vi "1.1 PID Squared .vi"(9 "2.1 PID Gains":T1={"P Gain"=0.25, "I Gain"=0.9999923706054688, "D Gain"=0.0, "P Gain - Exp"=2, "I Gain - Exp"=2, "D Gain - Exp"=2, "I Saturate"=0.25} {"I Saturate" format="%#_14g"; "P Gain" format="%.8f"; "I Gain" format="%.8f"; "D Gain" format="%.8f"}, 10 "Setpoint":i32, 11 "Encoder Value":i32) -> (0 "D Error":fxp<+/-,18,1> format="%.18g", 1 "I Error":fxp<+/-,64,46> format="%.32g", 2 "Analog Output":fxp<+/-,20,5> format="%.17g", 4 "Error":fxp<+/-,18,1> format="%.18g")   [LabVIEW 2010]
doc: "PID controll for FPGA (fixed point math) without the \"I\" or the \"D\""
uses:
  2-Low Neurons/2.1 PID Gains Typedef.ctl
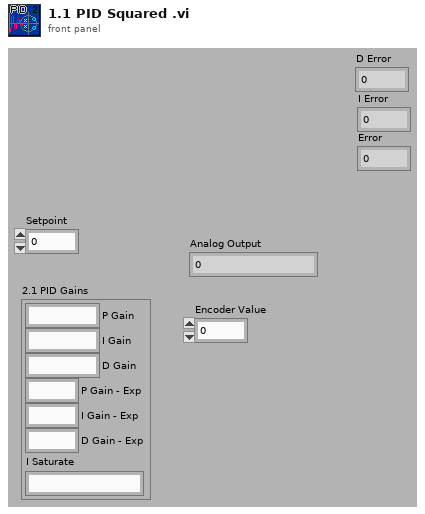
[diagram p1: front panel]
types:
  T1 = typedef "2.1 PID Gains Typedef.ctl" = cluster{"P Gain":fxp<+/-,18,1>, "I Gain":fxp<+/-,18,1>, "D Gain":fxp<+/-,18,1>, "P Gain - Exp":i8, "I Gain - Exp":i8, "D Gain - Exp":i8, "I Saturate":fxp<+/-,64,46>}
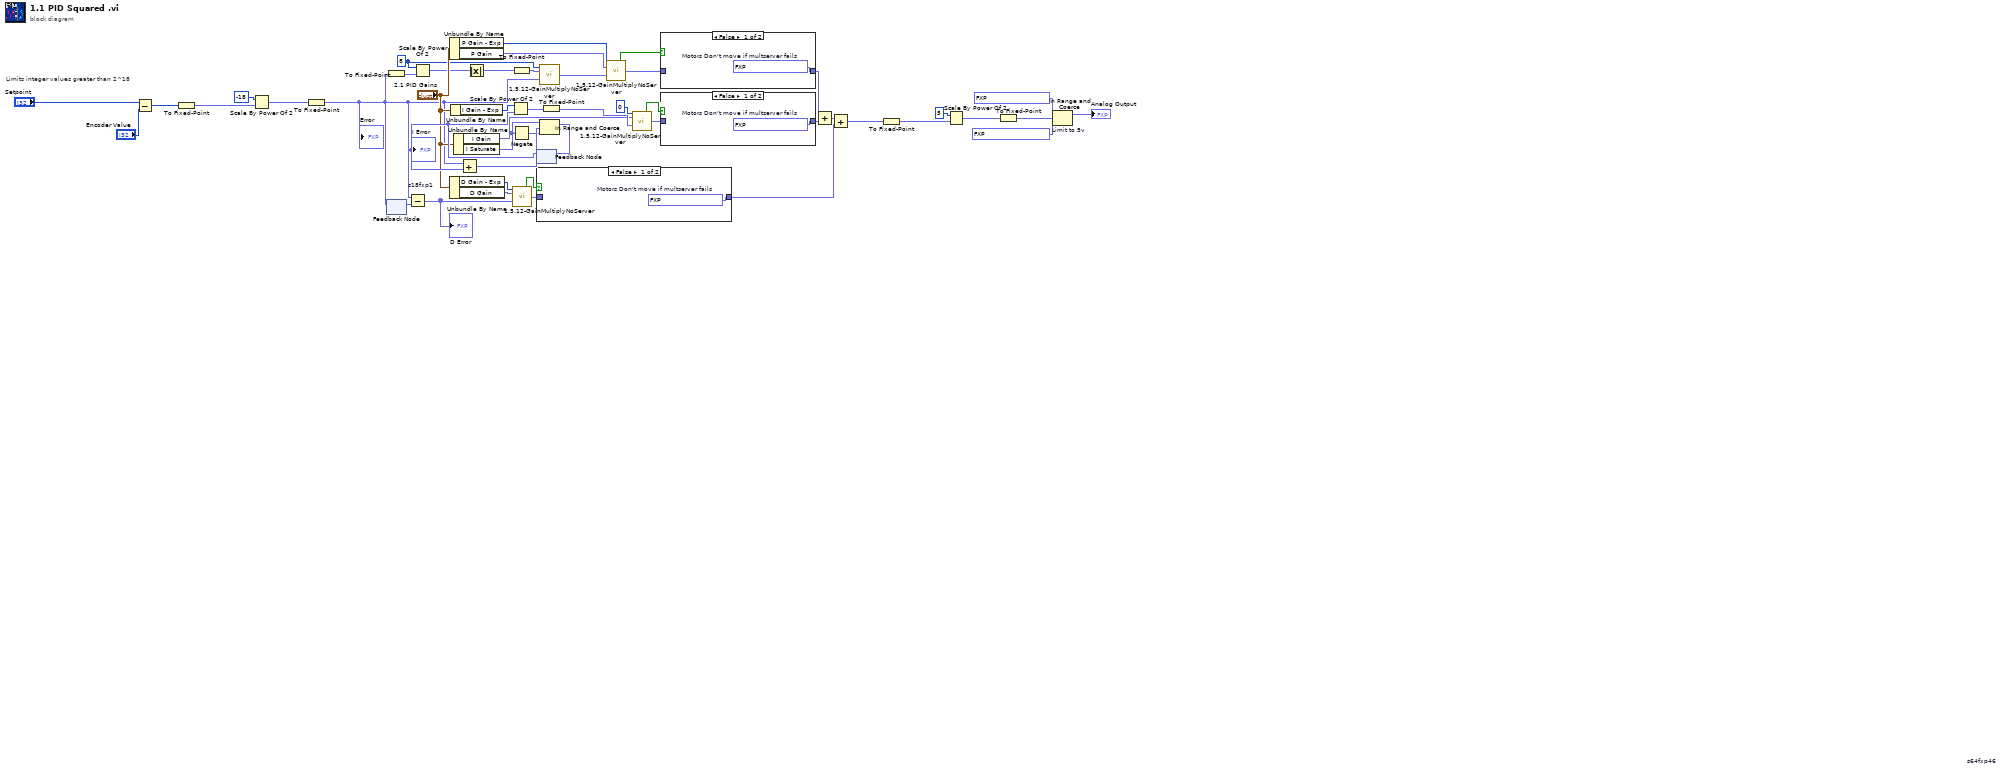
[diagram p0: block diagram]
diagram:
  w4 = i8 8 ("Gain Exponent")
  # "Limits integer values greater than 2^18"
  n1 = Subtract(x="Setpoint", y="Encoder Value") -> (x-y=w45:i32)
  n2 = To Fixed-Point(number=w45) -> (fixed-point=w44:fxp<+/-,34,18>)  [unwired: 1 in]
  n3 = Scale By Power Of 2(n=-18, x=w44) -> (x*2^n=w43:fxp<+/-,34,18>)
  n4 = To Fixed-Point(number=w43) -> (fixed-point=w6:fxp<+/-,18,1>)  [unwired: 1 in]
  "Error" <- w6
  n5 = To Fixed-Point(number=w6) -> (fixed-point=w5:fxp<+/-,54,18>)  [unwired: 1 in]
  n6 = feedback-in #1(w6) -> ()
  n7 = feedback #1() -> (w23:fxp<+/-,18,1>)  [unwired: 1 in]
  n8 = Subtract "s18fxp1"(x=w6, y=w23) -> (x-y=w22:fxp<+/-,18,1>)
  "D Error" <- w22
  n9 = Scale By Power Of 2(n=w4, x=w5) -> (x*2^n=w3:fxp<+/-,54,18>)
  n10 = Unbundle By Name("2.1 PID Gains") -> ("P Gain - Exp"=w18:i8, "P Gain"=w19:fxp<+/-,18,1>)
  n11 = Unbundle By Name("2.1 PID Gains") -> ("D Gain - Exp"=w15:i8, "D Gain"=w16:fxp<+/-,18,1>)
  n12 = Unbundle By Name("2.1 PID Gains") -> ("I Gain - Exp"=w25:i8)
  n13 = Unbundle By Name("2.1 PID Gains") -> ("I Gain"=w17:fxp<+/-,18,1>, "I Saturate"=w9:fxp<+/-,64,46>)
  n14 = Absolute Value(x=w3) -> (abs(x)=w2:fxp<+,54,18>)
  n15 = Negate(x=w9) -> (-x=w8:fxp<+/-,64,46>)
  n16 = To Fixed-Point(number=w2) -> (fixed-point=w1:fxp<+/-,18,1>)  [unwired: 1 in]
  n17 = call "1.5.12-GainMultiplyNoServer.vi"("Gain Exponent"=w15, "Gain"=w16, "Input"=w22) -> ("Result is Good"=w33:bool, "Output"=w36:fxp<+/-,18,1>)  [unwired: 11 in]
  n18 = feedback #2 "s64fxp46"() -> (w26:fxp<+/-,64,46>)  [unwired: 1 in]
  "I Error" <- w26
  n19 = Add(x=w6, y=w26) -> (x+y=w27:fxp<+/-,64,46>)
  n20 = Scale By Power Of 2(n=w25, x=w26) -> (x*2^n=w38:fxp<+/-,64,46>)
  n21 = case shown="False" w33 {
    tunnel: w36 -> [_ w50]
    tunnel: [w49 w50] -> w29
    frame False {
      w49 = fxp<+/-,18,1> 0.0  # Motors Don't move if multserver fails
    }
    frame True {
    }
  }
  n22 = call "1.5.12-GainMultiplyNoServer.vi"("Gain Exponent"=w4, "Gain"=w1, "Input"=w6) -> ("Output"=w7:fxp<+/-,18,1>)  [unwired: 11 in, 1 out]
  n23 = In Range and Coerce(upper limit=w9, x=w27, lower limit=w8) -> (coerced(x)=w10:fxp<+/-,64,46>)  [unwired: 1 out]
  n24 = feedback-in #2(w10) -> ()
  n25 = To Fixed-Point(number=w38) -> (fixed-point=w37:fxp<+/-,18,1>)  [unwired: 1 in]
  n26 = call "1.5.12-GainMultiplyNoServer.vi"("Gain Exponent"=w18, "Gain"=w19, "Input"=w7) -> ("Result is Good"=w40:bool, "Output"=w39:fxp<+/-,18,1>)  [unwired: 11 in]
  n27 = call "1.5.12-GainMultiplyNoServer.vi"("Gain Exponent"=i8 0, "Gain"=w17, "Input"=w37) -> ("Result is Good"=w34:bool, "Output"=w35:fxp<+/-,18,1>)  [unwired: 11 in]
  n28 = case shown="False" w40 {
    tunnel: w39 -> [_ w52]
    tunnel: [w51 w52] -> w32
    frame False {
      w51 = fxp<+/-,18,1> 0.0  # Motors Don't move if multserver fails
    }
    frame True {
    }
  }
  n29 = case shown="False" w34 {
    tunnel: w35 -> [_ w54]
    tunnel: [w53 w54] -> w31
    frame False {
      w53 = fxp<+/-,18,1> 0.0  # Motors Don't move if multserver fails
    }
    frame True {
    }
  }
  n30 = Add(x=w32, y=w31) -> (x+y=w30:fxp<+/-,18,1>)
  n31 = Add(x=w30, y=w29) -> (x+y=w28:fxp<+/-,18,1>)
  n32 = To Fixed-Point(number=w28) -> (fixed-point=w14:fxp<+/-,23,6>)  [unwired: 1 in]
  n33 = Scale By Power Of 2(n=5, x=w14) -> (x*2^n=w13:fxp<+/-,23,6>)
  n34 = To Fixed-Point(number=w13) -> (fixed-point=w11:fxp<+/-,20,5>)  [unwired: 1 in]
  n35 = In Range and Coerce "Limit to 5v"(upper limit=fxp<+/-,20,5> 5.0, x=w11, lower limit=fxp<+/-,20,5> -5.0 ("upper limit")) -> (coerced(x)=→"Analog Output":fxp<+/-,20,5>)  [unwired: 1 out]
